vi "Lab Panel V4.83.vi"() -> ()   [LabVIEW 2013] (continued)
                            n2023 = local read "TDMS LAB02-2"() -> (w3251:refnum<k34>)
                            n2024 = Build Array(w3248) -> (w3243:dbl[])
                            n2025 = Build Array(w3246) -> (w3242:dbl[])
                            n2026 = Build Array(w3253) -> (w3241:dbl[])
                            n2027 = Build Array(w3254) -> (w3240:dbl[])
                            n2028 = Build Array(w3249) -> (w3245:dbl[])
                            n2029 = Build Array(w3247) -> (w3244:dbl[])
                            n2030 = Build Array(w3252) -> (w3239:dbl[])
                            n2031 = Build Array("AMPS ON", "AMPS OFF", "VOLTS", "PF", "TEMP Live", "TEMP Neut", "CYCLE") -> (w3222:string[])
                            n2032 = Bundle By Name("Y"=w3245, "t0"=w3238) -> (w3237:waveform(dbl))  [unwired: 1 in]
                            n2033 = Bundle By Name("Y"=w3244, "t0"=w3238) -> (w3236:waveform(dbl))  [unwired: 1 in]
                            n2034 = Bundle By Name("Y"=w3243, "t0"=w3238) -> (w3235:waveform(dbl))  [unwired: 1 in]
                            n2035 = Bundle By Name("Y"=w3242, "t0"=w3238) -> (w3234:waveform(dbl))  [unwired: 1 in]
                            n2036 = Bundle By Name("Y"=w3241, "t0"=w3238) -> (w3233:waveform(dbl))  [unwired: 1 in]
                            n2037 = Bundle By Name("Y"=w3240, "t0"=w3238) -> (w3232:waveform(dbl))  [unwired: 1 in]
                            n2038 = Bundle By Name("Y"=w3239, "t0"=w3238) -> (w3231:waveform(dbl))  [unwired: 1 in]
                            n2039 = Build Array(w3237, w3236, w3235, w3234, w3233, w3232, w3231) -> (w3230:waveform(dbl)[])
                            n2040 = TDMS Write(0:w3251, 5:"TEST VALUES", 7:w3222, 9:w3230) -> (4:w3221:refnum<k34>, 6:w3220:string, 15:w3219:errorcluster)  [unwired: 2 in, 1 out]
                            n2041 = TDMS Write(0:w3221, 5:w3220, 7:"TIME", 9:w3217, 11:w3219) -> (15:w3216:errorcluster)  [unwired: 1 in, 3 out]
                            n2042 = local write "data file error"(w3216) -> ()
                          }
                        }
                      }
                    }
                  }
                }
              }
              frame #4 {
                n2043 = case shown="True" w3255 {
                  tunnel: w3259 -> [_ w3264]
                  tunnel: w3258 -> [_ w3263]
                  tunnel: w3257 -> [_ w3261]
                  tunnel: w3256 -> [_ w3260]
                  frame False {
                  }
                  frame True {
                    n2044 = local read "DISP LAB03-1"() -> (w3265:T4)
                    n2045 = local read "SIG LAB03-1"() -> (w3266:T2)
                    n2046 = local read "ON L03-1"() -> (w3262:cluster{"amps":dbl, "volts":dbl, "pf":dbl})
                    n2047 = Unbundle(w3266) -> ("AMPS"=w3272:dbl, "VOLTS"=w3270:dbl, "PF"=w3269:dbl, "Tmp Live"=w3268:dbl, "Tmp Neut"=w3271:dbl)
                    n2048 = Unbundle(w3265) -> ("CYCLE"=w3267:dbl)  [unwired: 2 out]
                    n2049 = stacked-sequence {
                      tunnel: w3272 -> [w3276 w3295]
                      tunnel: w3271 -> [_ w3294]
                      tunnel: w3270 -> [w3275 w3293]
                      tunnel: w3269 -> [w3274 w3292]
                      tunnel: w3268 -> [_ w3291]
                      tunnel: w3267 -> [_ w3290]
                      tunnel: w3264 -> [_ w3289]
                      tunnel: w3263 -> [w3277 _]
                      tunnel: w3262 -> [w3273 w3287]
                      tunnel: w3261 -> [_ w3288]
                      tunnel: w3260 -> [_ w3283]
                      frame #0 {
                        n2050 = case shown="True" w3277 {
                          tunnel: w3276 -> [_ w3282]
                          tunnel: w3275 -> [_ w3281]
                          tunnel: w3274 -> [_ w3280]
                          tunnel: w3273 -> [_ w3278]
                          frame False {
                          }
                          frame True {
                            n2051 = Bundle(cluster=w3278, "amps"=w3282, "volts"=w3281, "pf"=w3280) -> (w3279:cluster{"amps":dbl, "volts":dbl, "pf":dbl})
                            n2052 = local write "ON L03-1"(w3279) -> ()
                          }
                        }
                      }
                      frame #1 {
                        n2053 = Unbundle(w3287) -> ("amps"=w3286:dbl, "volts"=w3285:dbl, "pf"=w3284:dbl)
                        n2054 = case shown="True" w3288 {
                          tunnel: w3295 -> [_ w3327]
                          tunnel: w3294 -> [_ w3334]
                          tunnel: w3293 -> [_ _]
                          tunnel: w3292 -> [_ _]
                          tunnel: w3291 -> [_ w3333]
                          tunnel: w3290 -> [_ w3332]
                          tunnel: w3289 -> [_ w3297]
                          tunnel: w3286 -> [_ w3329]
                          tunnel: w3285 -> [_ w3328]
                          tunnel: w3284 -> [_ w3326]
                          tunnel: w3283 -> [_ w3318]
                          frame False {
                          }
                          frame True {
                            n2055 = local read "TDMS LAB03-1"() -> (w3331:refnum<k34>)
                            n2056 = Build Array(w3328) -> (w3323:dbl[])
                            n2057 = Build Array(w3326) -> (w3322:dbl[])
                            n2058 = Build Array(w3333) -> (w3321:dbl[])
                            n2059 = Build Array(w3334) -> (w3320:dbl[])
                            n2060 = Build Array(w3329) -> (w3325:dbl[])
                            n2061 = Build Array(w3327) -> (w3324:dbl[])
                            n2062 = Build Array(w3332) -> (w3319:dbl[])
                            n2063 = Build Array("AMPS ON", "AMPS OFF", "VOLTS", "PF", "TEMP Live", "TEMP Neut", "CYCLE") -> (w3302:string[])
                            n2064 = Bundle By Name("Y"=w3325, "t0"=w3318) -> (w3317:waveform(dbl))  [unwired: 1 in]
                            n2065 = Bundle By Name("Y"=w3324, "t0"=w3318) -> (w3316:waveform(dbl))  [unwired: 1 in]
                            n2066 = Bundle By Name("Y"=w3323, "t0"=w3318) -> (w3315:waveform(dbl))  [unwired: 1 in]
                            n2067 = Bundle By Name("Y"=w3322, "t0"=w3318) -> (w3314:waveform(dbl))  [unwired: 1 in]
                            n2068 = Bundle By Name("Y"=w3321, "t0"=w3318) -> (w3313:waveform(dbl))  [unwired: 1 in]
                            n2069 = Bundle By Name("Y"=w3320, "t0"=w3318) -> (w3312:waveform(dbl))  [unwired: 1 in]
                            n2070 = Bundle By Name("Y"=w3319, "t0"=w3318) -> (w3311:waveform(dbl))  [unwired: 1 in]
                            n2071 = Build Array(w3317, w3316, w3315, w3314, w3313, w3312, w3311) -> (w3310:waveform(dbl)[])
                            n2072 = TDMS Write(0:w3331, 5:"TEST VALUES", 7:w3302, 9:w3310) -> (4:w3301:refnum<k34>, 6:w3300:string, 15:w3299:errorcluster)  [unwired: 2 in, 1 out]
                            n2073 = TDMS Write(0:w3301, 5:w3300, 7:"TIME", 9:w3297, 11:w3299) -> (15:w3296:errorcluster)  [unwired: 1 in, 3 out]
                            n2074 = local write "data file error"(w3296) -> ()
                          }
                        }
                      }
                    }
                  }
                }
              }
              frame #5 {
                n2075 = case shown="True" w3335 {
                  tunnel: w3339 -> [_ w3344]
                  tunnel: w3338 -> [_ w3343]
                  tunnel: w3337 -> [_ w3341]
                  tunnel: w3336 -> [_ w3340]
                  frame False {
                  }
                  frame True {
                    n2076 = local read "DISP LAB03-2"() -> (w3345:T4)
                    n2077 = local read "SIG LAB03-2"() -> (w3346:T2)
                    n2078 = local read "ON L03-2"() -> (w3342:cluster{"amps":dbl, "volts":dbl, "pf":dbl})
                    n2079 = Unbundle(w3346) -> ("AMPS"=w3352:dbl, "VOLTS"=w3350:dbl, "PF"=w3349:dbl, "Tmp Live"=w3348:dbl, "Tmp Neut"=w3351:dbl)
                    n2080 = Unbundle(w3345) -> ("CYCLE"=w3347:dbl)  [unwired: 2 out]
                    n2081 = stacked-sequence {
                      tunnel: w3352 -> [w3356 w3375]
                      tunnel: w3351 -> [_ w3374]
                      tunnel: w3350 -> [w3355 w3373]
                      tunnel: w3349 -> [w3354 w3372]
                      tunnel: w3348 -> [_ w3371]
                      tunnel: w3347 -> [_ w3370]
                      tunnel: w3344 -> [_ w3369]
                      tunnel: w3343 -> [w3357 _]
                      tunnel: w3342 -> [w3353 w3367]
                      tunnel: w3341 -> [_ w3368]
                      tunnel: w3340 -> [_ w3363]
                      frame #0 {
                        n2082 = case shown="True" w3357 {
                          tunnel: w3356 -> [_ w3362]
                          tunnel: w3355 -> [_ w3361]
                          tunnel: w3354 -> [_ w3360]
                          tunnel: w3353 -> [_ w3358]
                          frame False {
                          }
                          frame True {
                            n2083 = Bundle(cluster=w3358, "amps"=w3362, "volts"=w3361, "pf"=w3360) -> (w3359:cluster{"amps":dbl, "volts":dbl, "pf":dbl})
                            n2084 = local write "ON L03-2"(w3359) -> ()
                          }
                        }
                      }
                      frame #1 {
                        n2085 = Unbundle(w3367) -> ("amps"=w3366:dbl, "volts"=w3365:dbl, "pf"=w3364:dbl)
                        n2086 = case shown="True" w3368 {
                          tunnel: w3375 -> [_ w3407]
                          tunnel: w3374 -> [_ w3414]
                          tunnel: w3373 -> [_ _]
                          tunnel: w3372 -> [_ _]
                          tunnel: w3371 -> [_ w3413]
                          tunnel: w3370 -> [_ w3412]
                          tunnel: w3369 -> [_ w3377]
                          tunnel: w3366 -> [_ w3409]
                          tunnel: w3365 -> [_ w3408]
                          tunnel: w3364 -> [_ w3406]
                          tunnel: w3363 -> [_ w3398]
                          frame False {
                          }
                          frame True {
                            n2087 = local read "TDMS LAB03-2"() -> (w3411:refnum<k34>)
                            n2088 = Build Array(w3408) -> (w3403:dbl[])
                            n2089 = Build Array(w3406) -> (w3402:dbl[])
                            n2090 = Build Array(w3413) -> (w3401:dbl[])
                            n2091 = Build Array(w3414) -> (w3400:dbl[])
                            n2092 = Build Array(w3409) -> (w3405:dbl[])
                            n2093 = Build Array(w3407) -> (w3404:dbl[])
                            n2094 = Build Array(w3412) -> (w3399:dbl[])
                            n2095 = Build Array("AMPS ON", "AMPS OFF", "VOLTS", "PF", "TEMP Live", "TEMP Neut", "CYCLE") -> (w3382:string[])
                            n2096 = Bundle By Name("Y"=w3405, "t0"=w3398) -> (w3397:waveform(dbl))  [unwired: 1 in]
                            n2097 = Bundle By Name("Y"=w3404, "t0"=w3398) -> (w3396:waveform(dbl))  [unwired: 1 in]
                            n2098 = Bundle By Name("Y"=w3403, "t0"=w3398) -> (w3395:waveform(dbl))  [unwired: 1 in]
                            n2099 = Bundle By Name("Y"=w3402, "t0"=w3398) -> (w3394:waveform(dbl))  [unwired: 1 in]
                            n2100 = Bundle By Name("Y"=w3401, "t0"=w3398) -> (w3393:waveform(dbl))  [unwired: 1 in]
                            n2101 = Bundle By Name("Y"=w3400, "t0"=w3398) -> (w3392:waveform(dbl))  [unwired: 1 in]
                            n2102 = Bundle By Name("Y"=w3399, "t0"=w3398) -> (w3391:waveform(dbl))  [unwired: 1 in]
                            n2103 = Build Array(w3397, w3396, w3395, w3394, w3393, w3392, w3391) -> (w3390:waveform(dbl)[])
                            n2104 = TDMS Write(0:w3411, 5:"TEST VALUES", 7:w3382, 9:w3390) -> (4:w3381:refnum<k34>, 6:w3380:string, 15:w3379:errorcluster)  [unwired: 2 in, 1 out]
                            n2105 = TDMS Write(0:w3381, 5:w3380, 7:"TIME", 9:w3377, 11:w3379) -> (15:w3376:errorcluster)  [unwired: 1 in, 3 out]
                            n2106 = local write "data file error"(w3376) -> ()
                          }
                        }
                      }
                    }
                  }
                }
              }
              frame #6 {
                n2107 = case shown="True" w3415 {
                  tunnel: w3419 -> [_ w3424]
                  tunnel: w3418 -> [_ w3423]
                  tunnel: w3417 -> [_ w3421]
                  tunnel: w3416 -> [_ w3420]
                  frame False {
                  }
                  frame True {
                    n2108 = local read "DISP LAB04-1"() -> (w3425:T4)
                    n2109 = local read "SIG LAB04-1"() -> (w3426:T2)
                    n2110 = local read "ON L04-1"() -> (w3422:cluster{"amps":dbl, "volts":dbl, "pf":dbl})
                    n2111 = Unbundle(w3426) -> ("AMPS"=w3432:dbl, "VOLTS"=w3430:dbl, "PF"=w3429:dbl, "Tmp Live"=w3428:dbl, "Tmp Neut"=w3431:dbl)
                    n2112 = Unbundle(w3425) -> ("CYCLE"=w3427:dbl)  [unwired: 2 out]
                    n2113 = stacked-sequence {
                      tunnel: w3432 -> [w3436 w3455]
                      tunnel: w3431 -> [_ w3454]
                      tunnel: w3430 -> [w3435 w3453]
                      tunnel: w3429 -> [w3434 w3452]
                      tunnel: w3428 -> [_ w3451]
                      tunnel: w3427 -> [_ w3450]
                      tunnel: w3424 -> [_ w3449]
                      tunnel: w3423 -> [w3437 _]
                      tunnel: w3422 -> [w3433 w3447]
                      tunnel: w3421 -> [_ w3448]
                      tunnel: w3420 -> [_ w3443]
                      frame #0 {
                        n2114 = case shown="True" w3437 {
                          tunnel: w3436 -> [_ w3442]
                          tunnel: w3435 -> [_ w3441]
                          tunnel: w3434 -> [_ w3440]
                          tunnel: w3433 -> [_ w3438]
                          frame False {
                          }
                          frame True {
                            n2115 = Bundle(cluster=w3438, "amps"=w3442, "volts"=w3441, "pf"=w3440) -> (w3439:cluster{"amps":dbl, "volts":dbl, "pf":dbl})
                            n2116 = local write "ON L04-1"(w3439) -> ()
                          }
                        }
                      }
                      frame #1 {
                        n2117 = Unbundle(w3447) -> ("amps"=w3446:dbl, "volts"=w3445:dbl, "pf"=w3444:dbl)
                        n2118 = case shown="True" w3448 {
                          tunnel: w3455 -> [_ w3487]
                          tunnel: w3454 -> [_ w3494]
                          tunnel: w3453 -> [_ _]
                          tunnel: w3452 -> [_ _]
                          tunnel: w3451 -> [_ w3493]
                          tunnel: w3450 -> [_ w3492]
                          tunnel: w3449 -> [_ w3457]
                          tunnel: w3446 -> [_ w3489]
                          tunnel: w3445 -> [_ w3488]
                          tunnel: w3444 -> [_ w3486]
                          tunnel: w3443 -> [_ w3478]
                          frame False {
                          }
                          frame True {
                            n2119 = local read "TDMS LAB04-1"() -> (w3491:refnum<k34>)
                            n2120 = Build Array(w3488) -> (w3483:dbl[])
                            n2121 = Build Array(w3486) -> (w3482:dbl[])
                            n2122 = Build Array(w3493) -> (w3481:dbl[])
                            n2123 = Build Array(w3494) -> (w3480:dbl[])
                            n2124 = Build Array(w3489) -> (w3485:dbl[])
                            n2125 = Build Array(w3487) -> (w3484:dbl[])
                            n2126 = Build Array(w3492) -> (w3479:dbl[])
                            n2127 = Build Array("AMPS ON", "AMPS OFF", "VOLTS", "PF", "TEMP Live", "TEMP Neut", "CYCLE") -> (w3462:string[])
                            n2128 = Bundle By Name("Y"=w3485, "t0"=w3478) -> (w3477:waveform(dbl))  [unwired: 1 in]
                            n2129 = Bundle By Name("Y"=w3484, "t0"=w3478) -> (w3476:waveform(dbl))  [unwired: 1 in]
                            n2130 = Bundle By Name("Y"=w3483, "t0"=w3478) -> (w3475:waveform(dbl))  [unwired: 1 in]
                            n2131 = Bundle By Name("Y"=w3482, "t0"=w3478) -> (w3474:waveform(dbl))  [unwired: 1 in]
                            n2132 = Bundle By Name("Y"=w3481, "t0"=w3478) -> (w3473:waveform(dbl))  [unwired: 1 in]
                            n2133 = Bundle By Name("Y"=w3480, "t0"=w3478) -> (w3472:waveform(dbl))  [unwired: 1 in]
                            n2134 = Bundle By Name("Y"=w3479, "t0"=w3478) -> (w3471:waveform(dbl))  [unwired: 1 in]
                            n2135 = Build Array(w3477, w3476, w3475, w3474, w3473, w3472, w3471) -> (w3470:waveform(dbl)[])
                            n2136 = TDMS Write(0:w3491, 5:"TEST VALUES", 7:w3462, 9:w3470) -> (4:w3461:refnum<k34>, 6:w3460:string, 15:w3459:errorcluster)  [unwired: 2 in, 1 out]
                            n2137 = TDMS Write(0:w3461, 5:w3460, 7:"TIME", 9:w3457, 11:w3459) -> (15:w3456:errorcluster)  [unwired: 1 in, 3 out]
                            n2138 = local write "data file error"(w3456) -> ()
                          }
                        }
                      }
                    }
                  }
                }
              }
              frame #7 {
                n2139 = case shown="True" w3495 {
                  tunnel: w3499 -> [_ w3504]
                  tunnel: w3498 -> [_ w3503]
                  tunnel: w3497 -> [_ w3501]
                  tunnel: w3496 -> [_ w3500]
                  frame False {
                  }
                  frame True {
                    n2140 = local read "DISP LAB04-2"() -> (w3505:T4)
                    n2141 = local read "SIG LAB04-2"() -> (w3506:T2)
                    n2142 = local read "ON L04-2"() -> (w3502:cluster{"amps":dbl, "volts":dbl, "pf":dbl})
                    n2143 = Unbundle(w3506) -> ("AMPS"=w3512:dbl, "VOLTS"=w3510:dbl, "PF"=w3509:dbl, "Tmp Live"=w3508:dbl, "Tmp Neut"=w3511:dbl)
                    n2144 = Unbundle(w3505) -> ("CYCLE"=w3507:dbl)  [unwired: 2 out]
                    n2145 = stacked-sequence {
                      tunnel: w3512 -> [w3516 w3535]
                      tunnel: w3511 -> [_ w3534]
                      tunnel: w3510 -> [w3515 w3533]
                      tunnel: w3509 -> [w3514 w3532]
                      tunnel: w3508 -> [_ w3531]
                      tunnel: w3507 -> [_ w3530]
                      tunnel: w3504 -> [_ w3529]
                      tunnel: w3503 -> [w3517 _]
                      tunnel: w3502 -> [w3513 w3527]
                      tunnel: w3501 -> [_ w3528]
                      tunnel: w3500 -> [_ w3523]
                      frame #0 {
                        n2146 = case shown="True" w3517 {
                          tunnel: w3516 -> [_ w3522]
                          tunnel: w3515 -> [_ w3521]
                          tunnel: w3514 -> [_ w3520]
                          tunnel: w3513 -> [_ w3518]
                          frame False {
                          }
                          frame True {
                            n2147 = Bundle(cluster=w3518, "amps"=w3522, "volts"=w3521, "pf"=w3520) -> (w3519:cluster{"amps":dbl, "volts":dbl, "pf":dbl})
                            n2148 = local write "ON L04-2"(w3519) -> ()
                          }
                        }
                      }
                      frame #1 {
                        n2149 = Unbundle(w3527) -> ("amps"=w3526:dbl, "volts"=w3525:dbl, "pf"=w3524:dbl)
                        n2150 = case shown="True" w3528 {
                          tunnel: w3535 -> [_ w3567]
                          tunnel: w3534 -> [_ w3574]
                          tunnel: w3533 -> [_ _]
                          tunnel: w3532 -> [_ _]
                          tunnel: w3531 -> [_ w3573]
                          tunnel: w3530 -> [_ w3572]
                          tunnel: w3529 -> [_ w3537]
                          tunnel: w3526 -> [_ w3569]
                          tunnel: w3525 -> [_ w3568]
                          tunnel: w3524 -> [_ w3566]
                          tunnel: w3523 -> [_ w3558]
                          frame False {
                          }
                          frame True {
                            n2151 = local read "TDMS LAB04-2"() -> (w3571:refnum<k34>)
                            n2152 = Build Array(w3568) -> (w3563:dbl[])
                            n2153 = Build Array(w3566) -> (w3562:dbl[])
                            n2154 = Build Array(w3573) -> (w3561:dbl[])
                            n2155 = Build Array(w3574) -> (w3560:dbl[])
                            n2156 = Build Array(w3569) -> (w3565:dbl[])
                            n2157 = Build Array(w3567) -> (w3564:dbl[])
                            n2158 = Build Array(w3572) -> (w3559:dbl[])
                            n2159 = Build Array("AMPS ON", "AMPS OFF", "VOLTS", "PF", "TEMP Live", "TEMP Neut", "CYCLE") -> (w3542:string[])
                            n2160 = Bundle By Name("Y"=w3565, "t0"=w3558) -> (w3557:waveform(dbl))  [unwired: 1 in]
                            n2161 = Bundle By Name("Y"=w3564, "t0"=w3558) -> (w3556:waveform(dbl))  [unwired: 1 in]
                            n2162 = Bundle By Name("Y"=w3563, "t0"=w3558) -> (w3555:waveform(dbl))  [unwired: 1 in]
                            n2163 = Bundle By Name("Y"=w3562, "t0"=w3558) -> (w3554:waveform(dbl))  [unwired: 1 in]
                            n2164 = Bundle By Name("Y"=w3561, "t0"=w3558) -> (w3553:waveform(dbl))  [unwired: 1 in]
                            n2165 = Bundle By Name("Y"=w3560, "t0"=w3558) -> (w3552:waveform(dbl))  [unwired: 1 in]
                            n2166 = Bundle By Name("Y"=w3559, "t0"=w3558) -> (w3551:waveform(dbl))  [unwired: 1 in]
                            n2167 = Build Array(w3557, w3556, w3555, w3554, w3553, w3552, w3551) -> (w3550:waveform(dbl)[])
                            n2168 = TDMS Write(0:w3571, 5:"TEST VALUES", 7:w3542, 9:w3550) -> (4:w3541:refnum<k34>, 6:w3540:string, 15:w3539:errorcluster)  [unwired: 2 in, 1 out]
                            n2169 = TDMS Write(0:w3541, 5:w3540, 7:"TIME", 9:w3537, 11:w3539) -> (15:w3536:errorcluster)  [unwired: 1 in, 3 out]
                            n2170 = local write "data file error"(w3536) -> ()
                          }
                        }
                      }
                    }
                  }
                }
              }
              frame #8 {
                n2171 = case shown="True" w3575 {
                  tunnel: w3579 -> [_ w3584]
                  tunnel: w3578 -> [_ w3583]
                  tunnel: w3577 -> [_ w3581]
                  tunnel: w3576 -> [_ w3580]
                  frame False {
                  }
                  frame True {
                    n2172 = local read "DISP LAB05-1"() -> (w3585:T4)
                    n2173 = local read "SIG LAB05-1"() -> (w3586:T2)
                    n2174 = local read "ON L05-1"() -> (w3582:cluster{"amps":dbl, "volts":dbl, "pf":dbl})
                    n2175 = Unbundle(w3586) -> ("AMPS"=w3592:dbl, "VOLTS"=w3590:dbl, "PF"=w3589:dbl, "Tmp Live"=w3588:dbl, "Tmp Neut"=w3591:dbl)
                    n2176 = Unbundle(w3585) -> ("CYCLE"=w3587:dbl)  [unwired: 2 out]
                    n2177 = stacked-sequence {
                      tunnel: w3592 -> [w3596 w3615]
                      tunnel: w3591 -> [_ w3614]
                      tunnel: w3590 -> [w3595 w3613]
                      tunnel: w3589 -> [w3594 w3612]
                      tunnel: w3588 -> [_ w3611]
                      tunnel: w3587 -> [_ w3610]
                      tunnel: w3584 -> [_ w3609]
                      tunnel: w3583 -> [w3597 _]
                      tunnel: w3582 -> [w3593 w3607]
                      tunnel: w3581 -> [_ w3608]
                      tunnel: w3580 -> [_ w3603]
                      frame #0 {
                        n2178 = case shown="True" w3597 {
                          tunnel: w3596 -> [_ w3602]
                          tunnel: w3595 -> [_ w3601]
                          tunnel: w3594 -> [_ w3600]
                          tunnel: w3593 -> [_ w3598]
                          frame False {
                          }
                          frame True {
                            n2179 = Bundle(cluster=w3598, "amps"=w3602, "volts"=w3601, "pf"=w3600) -> (w3599:cluster{"amps":dbl, "volts":dbl, "pf":dbl})
                            n2180 = local write "ON L05-1"(w3599) -> ()
                          }
                        }
                      }
                      frame #1 {
                        n2181 = Unbundle(w3607) -> ("amps"=w3606:dbl, "volts"=w3605:dbl, "pf"=w3604:dbl)
                        n2182 = case shown="True" w3608 {
                          tunnel: w3615 -> [_ w3647]
                          tunnel: w3614 -> [_ w3654]
                          tunnel: w3613 -> [_ _]
                          tunnel: w3612 -> [_ _]
                          tunnel: w3611 -> [_ w3653]
                          tunnel: w3610 -> [_ w3652]
                          tunnel: w3609 -> [_ w3617]
                          tunnel: w3606 -> [_ w3649]
                          tunnel: w3605 -> [_ w3648]
                          tunnel: w3604 -> [_ w3646]
                          tunnel: w3603 -> [_ w3638]
                          frame False {
                          }
                          frame True {
                            n2183 = local read "TDMS LAB05-1"() -> (w3651:refnum<k34>)
                            n2184 = Build Array(w3648) -> (w3643:dbl[])
                            n2185 = Build Array(w3646) -> (w3642:dbl[])
                            n2186 = Build Array(w3653) -> (w3641:dbl[])
                            n2187 = Build Array(w3654) -> (w3640:dbl[])
                            n2188 = Build Array(w3649) -> (w3645:dbl[])
                            n2189 = Build Array(w3647) -> (w3644:dbl[])
                            n2190 = Build Array(w3652) -> (w3639:dbl[])
                            n2191 = Build Array("AMPS ON", "AMPS OFF", "VOLTS", "PF", "TEMP Live", "TEMP Neut", "CYCLE") -> (w3622:string[])
                            n2192 = Bundle By Name("Y"=w3645, "t0"=w3638) -> (w3637:waveform(dbl))  [unwired: 1 in]
                            n2193 = Bundle By Name("Y"=w3644, "t0"=w3638) -> (w3636:waveform(dbl))  [unwired: 1 in]
                            n2194 = Bundle By Name("Y"=w3643, "t0"=w3638) -> (w3635:waveform(dbl))  [unwired: 1 in]
                            n2195 = Bundle By Name("Y"=w3642, "t0"=w3638) -> (w3634:waveform(dbl))  [unwired: 1 in]
                            n2196 = Bundle By Name("Y"=w3641, "t0"=w3638) -> (w3633:waveform(dbl))  [unwired: 1 in]
                            n2197 = Bundle By Name("Y"=w3640, "t0"=w3638) -> (w3632:waveform(dbl))  [unwired: 1 in]
                            n2198 = Bundle By Name("Y"=w3639, "t0"=w3638) -> (w3631:waveform(dbl))  [unwired: 1 in]
                            n2199 = Build Array(w3637, w3636, w3635, w3634, w3633, w3632, w3631) -> (w3630:waveform(dbl)[])
                            n2200 = TDMS Write(0:w3651, 5:"TEST VALUES", 7:w3622, 9:w3630) -> (4:w3621:refnum<k34>, 6:w3620:string, 15:w3619:errorcluster)  [unwired: 2 in, 1 out]
                            n2201 = TDMS Write(0:w3621, 5:w3620, 7:"TIME", 9:w3617, 11:w3619) -> (15:w3616:errorcluster)  [unwired: 1 in, 3 out]
                            n2202 = local write "data file error"(w3616) -> ()
                          }
                        }
                      }
                    }
                  }
                }
              }
              frame #9 {
                n2203 = case shown="True" w3655 {
                  tunnel: w3659 -> [_ w3664]
                  tunnel: w3658 -> [_ w3663]
                  tunnel: w3657 -> [_ w3661]
                  tunnel: w3656 -> [_ w3660]
                  frame False {
                  }
                  frame True {
                    n2204 = local read "DISP LAB05-2"() -> (w3665:T4)
                    n2205 = local read "SIG LAB05-2"() -> (w3666:T2)
                    n2206 = local read "ON L05-2"() -> (w3662:cluster{"amps":dbl, "volts":dbl, "pf":dbl})
                    n2207 = Unbundle(w3666) -> ("AMPS"=w3672:dbl, "VOLTS"=w3670:dbl, "PF"=w3669:dbl, "Tmp Live"=w3668:dbl, "Tmp Neut"=w3671:dbl)
                    n2208 = Unbundle(w3665) -> ("CYCLE"=w3667:dbl)  [unwired: 2 out]
                    n2209 = stacked-sequence {
                      tunnel: w3672 -> [w3676 w3695]
                      tunnel: w3671 -> [_ w3694]
                      tunnel: w3670 -> [w3675 w3693]
                      tunnel: w3669 -> [w3674 w3692]
                      tunnel: w3668 -> [_ w3691]
                      tunnel: w3667 -> [_ w3690]
                      tunnel: w3664 -> [_ w3689]
                      tunnel: w3663 -> [w3677 _]
                      tunnel: w3662 -> [w3673 w3687]
                      tunnel: w3661 -> [_ w3688]
                      tunnel: w3660 -> [_ w3683]
                      frame #0 {
                        n2210 = case shown="True" w3677 {
                          tunnel: w3676 -> [_ w3682]
                          tunnel: w3675 -> [_ w3681]
                          tunnel: w3674 -> [_ w3680]
                          tunnel: w3673 -> [_ w3678]
                          frame False {
                          }
                          frame True {
                            n2211 = Bundle(cluster=w3678, "amps"=w3682, "volts"=w3681, "pf"=w3680) -> (w3679:cluster{"amps":dbl, "volts":dbl, "pf":dbl})
                            n2212 = local write "ON L05-2"(w3679) -> ()
                          }
                        }
                      }
                      frame #1 {
                        n2213 = Unbundle(w3687) -> ("amps"=w3686:dbl, "volts"=w3685:dbl, "pf"=w3684:dbl)
                        n2214 = case shown="True" w3688 {
                          tunnel: w3695 -> [_ w3727]
                          tunnel: w3694 -> [_ w3734]
                          tunnel: w3693 -> [_ _]
                          tunnel: w3692 -> [_ _]
                          tunnel: w3691 -> [_ w3733]
                          tunnel: w3690 -> [_ w3732]
                          tunnel: w3689 -> [_ w3697]
                          tunnel: w3686 -> [_ w3729]
                          tunnel: w3685 -> [_ w3728]
                          tunnel: w3684 -> [_ w3726]
                          tunnel: w3683 -> [_ w3718]
                          frame False {
                          }
                          frame True {
                            n2215 = local read "TDMS LAB05-2"() -> (w3731:refnum<k34>)
                            n2216 = Build Array(w3728) -> (w3723:dbl[])
                            n2217 = Build Array(w3726) -> (w3722:dbl[])
                            n2218 = Build Array(w3733) -> (w3721:dbl[])
                            n2219 = Build Array(w3734) -> (w3720:dbl[])
                            n2220 = Build Array(w3729) -> (w3725:dbl[])
                            n2221 = Build Array(w3727) -> (w3724:dbl[])
                            n2222 = Build Array(w3732) -> (w3719:dbl[])
                            n2223 = Build Array("AMPS ON", "AMPS OFF", "VOLTS", "PF", "TEMP Live", "TEMP Neut", "CYCLE") -> (w3702:string[])
                            n2224 = Bundle By Name("Y"=w3725, "t0"=w3718) -> (w3717:waveform(dbl))  [unwired: 1 in]
                            n2225 = Bundle By Name("Y"=w3724, "t0"=w3718) -> (w3716:waveform(dbl))  [unwired: 1 in]
                            n2226 = Bundle By Name("Y"=w3723, "t0"=w3718) -> (w3715:waveform(dbl))  [unwired: 1 in]
                            n2227 = Bundle By Name("Y"=w3722, "t0"=w3718) -> (w3714:waveform(dbl))  [unwired: 1 in]
                            n2228 = Bundle By Name("Y"=w3721, "t0"=w3718) -> (w3713:waveform(dbl))  [unwired: 1 in]
                            n2229 = Bundle By Name("Y"=w3720, "t0"=w3718) -> (w3712:waveform(dbl))  [unwired: 1 in]
                            n2230 = Bundle By Name("Y"=w3719, "t0"=w3718) -> (w3711:waveform(dbl))  [unwired: 1 in]
                            n2231 = Build Array(w3717, w3716, w3715, w3714, w3713, w3712, w3711) -> (w3710:waveform(dbl)[])
                            n2232 = TDMS Write(0:w3731, 5:"TEST VALUES", 7:w3702, 9:w3710) -> (4:w3701:refnum<k34>, 6:w3700:string, 15:w3699:errorcluster)  [unwired: 2 in, 1 out]
                            n2233 = TDMS Write(0:w3701, 5:w3700, 7:"TIME", 9:w3697, 11:w3699) -> (15:w3696:errorcluster)  [unwired: 1 in, 3 out]
                            n2234 = local write "data file error"(w3696) -> ()
                          }
                        }
                      }
                    }
                  }
                }
              }
            }
          }
          frame #13 {
            # "display test values on chart"
            n2235 = case shown="\"OFF CYCLE\"" "Select  Cycle" {
              tunnel: [1 w3740] -> w3736
              frame "ON CYCLE", Default {
              }
              frame "OFF CYCLE" {
                n2236 = local read "on loops"() -> (w3742:dbl)
                n2237 = Add(x=w3742, y=2) -> (x+y=w3740:dbl)
              }
            }
            n2238 = local read "jig cycle"() -> (w3738:dbl)
            n2239 = Equal?(x=w3738, y=w3736) -> (x = y?=w3735:bool)
            "graph flag" <- w3735
            n2240 = global write "Global display 3.vi" "graph flag"(w3735) -> ()
            n2241 = case shown="True" w3735 {
              frame False {
              }
              frame True {
                n2242 = local read "SIG LAB05-1"() -> (w3784:T2)
                n2243 = local read "SIG LAB04-2"() -> (w3785:T2)
                n2244 = local read "SIG LAB05-2"() -> (w3783:T2)
                n2245 = local read "SIG LAB04-1"() -> (w3786:T2)
                n2246 = local read "SIG LAB03-1"() -> (w3788:T2)
                n2247 = local read "SIG LAB03-2"() -> (w3787:T2)
                n2248 = local read "SIG LAB01-1"() -> (w3792:T2)
                n2249 = local read "SIG LAB02-2"() -> (w3789:T2)
                n2250 = local read "SIG LAB02-1"() -> (w3790:T2)
                n2251 = local read "SIG LAB01-2"() -> (w3791:T2)
                n2252 = Unbundle(w3785) -> ("AMPS"=w3775:dbl, "VOLTS"=w3765:dbl, "Tmp Live"=w3755:dbl, "Tmp Neut"=w3745:dbl)  [unwired: 1 out]
                n2253 = Unbundle(w3784) -> ("AMPS"=w3774:dbl, "VOLTS"=w3764:dbl, "Tmp Live"=w3754:dbl, "Tmp Neut"=w3744:dbl)  [unwired: 1 out]
                n2254 = Unbundle(w3783) -> ("AMPS"=w3773:dbl, "VOLTS"=w3763:dbl, "Tmp Live"=w3753:dbl, "Tmp Neut"=w3743:dbl)  [unwired: 1 out]
                n2255 = Unbundle(w3786) -> ("AMPS"=w3776:dbl, "VOLTS"=w3766:dbl, "Tmp Live"=w3756:dbl, "Tmp Neut"=w3746:dbl)  [unwired: 1 out]
                n2256 = Unbundle(w3787) -> ("AMPS"=w3777:dbl, "VOLTS"=w3767:dbl, "Tmp Live"=w3757:dbl, "Tmp Neut"=w3747:dbl)  [unwired: 1 out]
                n2257 = Unbundle(w3788) -> ("AMPS"=w3778:dbl, "VOLTS"=w3768:dbl, "Tmp Live"=w3758:dbl, "Tmp Neut"=w3748:dbl)  [unwired: 1 out]
                n2258 = Unbundle(w3789) -> ("AMPS"=w3779:dbl, "VOLTS"=w3769:dbl, "Tmp Live"=w3759:dbl, "Tmp Neut"=w3749:dbl)  [unwired: 1 out]
                n2259 = Unbundle(w3790) -> ("AMPS"=w3780:dbl, "VOLTS"=w3770:dbl, "Tmp Live"=w3760:dbl, "Tmp Neut"=w3750:dbl)  [unwired: 1 out]
                n2260 = Unbundle(w3792) -> ("AMPS"=w3782:dbl, "VOLTS"=w3772:dbl, "Tmp Live"=w3762:dbl, "Tmp Neut"=w3752:dbl)  [unwired: 1 out]
                n2261 = Unbundle(w3791) -> ("AMPS"=w3781:dbl, "VOLTS"=w3771:dbl, "Tmp Live"=w3761:dbl, "Tmp Neut"=w3751:dbl)  [unwired: 1 out]
                n2262 = stacked-sequence {
                  tunnel: w3782 -> [w3803 _ _ _ _]
                  tunnel: w3781 -> [w3802 _ _ _ _]
                  tunnel: w3780 -> [w3801 _ _ _ _]
                  tunnel: w3779 -> [w3800 _ _ _ _]
                  tunnel: w3778 -> [w3799 _ _ _ _]
                  tunnel: w3777 -> [w3798 _ _ _ _]
                  tunnel: w3776 -> [w3797 _ _ _ _]
                  tunnel: w3775 -> [w3796 _ _ _ _]
                  tunnel: w3774 -> [w3795 _ _ _ _]
                  tunnel: w3773 -> [w3794 _ _ _ _]
                  tunnel: w3772 -> [_ w3814 _ _ _]
                  tunnel: w3771 -> [_ w3813 _ _ _]
                  tunnel: w3770 -> [_ w3812 _ _ _]
                  tunnel: w3769 -> [_ w3811 _ _ _]
                  tunnel: w3768 -> [_ w3810 _ _ _]
                  tunnel: w3767 -> [_ w3809 _ _ _]
                  tunnel: w3766 -> [_ w3808 _ _ _]
                  tunnel: w3765 -> [_ w3807 _ _ _]
                  tunnel: w3764 -> [_ w3806 _ _ _]
                  tunnel: w3763 -> [_ w3805 _ _ _]
                  tunnel: w3762 -> [_ _ w3825 _ _]
                  tunnel: w3761 -> [_ _ w3824 _ _]
                  tunnel: w3760 -> [_ _ w3823 _ _]
                  tunnel: w3759 -> [_ _ w3822 _ _]
                  tunnel: w3758 -> [_ _ w3821 _ _]
                  tunnel: w3757 -> [_ _ w3820 _ _]
                  tunnel: w3756 -> [_ _ w3819 _ _]
                  tunnel: w3755 -> [_ _ w3818 _ _]
                  tunnel: w3754 -> [_ _ w3817 _ _]
                  tunnel: w3753 -> [_ _ w3816 _ _]
                  tunnel: w3752 -> [_ _ _ w3836 _]
                  tunnel: w3751 -> [_ _ _ w3835 _]
                  tunnel: w3750 -> [_ _ _ w3834 _]
                  tunnel: w3749 -> [_ _ _ w3833 _]
                  tunnel: w3748 -> [_ _ _ w3832 _]
                  tunnel: w3747 -> [_ _ _ w3831 _]
                  tunnel: w3746 -> [_ _ _ w3830 _]
                  tunnel: w3745 -> [_ _ _ w3829 _]
                  tunnel: w3744 -> [_ _ _ w3828 _]
                  tunnel: w3743 -> [_ _ _ w3827 _]
                  frame #0 {
                    n2263 = Merge Signals(w3803, w3802, w3801, w3800, w3799, w3798, w3797, w3796, w3795, w3794) -> (→"TEST AMPS CHART":dynamicdata)
                  }
                  frame #1 {
                    n2264 = Merge Signals(w3814, w3813, w3812, w3811, w3810, w3809, w3808, w3807, w3806, w3805) -> (→"TEST VOLTS CHART":dynamicdata)
                  }
                  frame #2 {
                    n2265 = Merge Signals(w3825, w3824, w3823, w3822, w3821, w3820, w3819, w3818, w3817, w3816) -> (→"TEMPERATURE (L) CHART":dynamicdata)
                  }
                  frame #3 {
                    n2266 = Merge Signals(w3836, w3835, w3834, w3833, w3832, w3831, w3830, w3829, w3828, w3827) -> (→"TEMPERATURE (N) CHART":dynamicdata)
                  }
                  frame #4 {
                    n2267 = local read "TEMPERATURE (N) CHART"() -> (w3837:dynamicdata)
                    n2268 = local read "TEMPERATURE (L) CHART"() -> (w3838:dynamicdata)
                    n2269 = local read "TEST VOLTS CHART"() -> (w3839:dynamicdata)
                    n2270 = local read "TEST AMPS CHART"() -> (w3840:dynamicdata)
                    n2271 = global write "Global display 3.vi" "graph temp N"(w3837) -> ()
                    n2272 = global write "Global display 3.vi" "graph temp L"(w3838) -> ()
                    n2273 = global write "Global display 3.vi" "graph volts"(w3839) -> ()
                    n2274 = global write "Global display 3.vi" "graph amps"(w3840) -> ()
                  }
                }
              }
            }
          }
          frame #14 {
            # "check for amps fail"
            # "check for cycle test & temperature rise fail conditions"
            n2275 = local read "on loops"() -> (w3867:dbl)
            n2276 = local read "jig cycle"() -> (w3864:dbl)
            n2277 = local read "jig cycle"() -> (w3869:dbl)
            n2278 = Add(x=w3867, y=3.0) -> (x+y=w3865:dbl)
            n2279 = Equal?(x=w3864, y=w3865) -> (x = y?=w3860:bool)
            n2280 = local read "Fail Loops"() -> (w3841:dbl)
            n2281 = Equal?(x=w3869, y=1.0) -> (x = y?=w3862:bool)
            n2282 = global write "Global 1.vi" "fail count"(w3841) -> ()
            n2283 = stacked-sequence {
              tunnel: w3863 -> [w3872 _ _ _ _ _ _ _ _ _]
              tunnel: w3862 -> [w3873 w3893 w3913 w3933 w3953 w3973 w3993 w4013 w4033 w4053]
              tunnel: w3861 -> [w3870 _ _ _ _ _ _ _ _ _]
              tunnel: w3860 -> [w3871 w3892 w3912 w3932 w3952 w3972 w3992 w4012 w4032 w4052]
              tunnel: w3859 -> [_ w3891 _ _ _ _ _ _ _ _]
              tunnel: w3858 -> [_ w3890 _ _ _ _ _ _ _ _]
              tunnel: w3857 -> [_ _ w3911 _ _ _ _ _ _ _]
              tunnel: w3856 -> [_ _ w3910 _ _ _ _ _ _ _]
              tunnel: w3855 -> [_ _ _ w3931 _ _ _ _ _ _]
              tunnel: w3854 -> [_ _ _ w3930 _ _ _ _ _ _]
              tunnel: w3853 -> [_ _ _ _ w3951 _ _ _ _ _]
              tunnel: w3852 -> [_ _ _ _ w3950 _ _ _ _ _]
              tunnel: w3851 -> [_ _ _ _ _ w3971 _ _ _ _]
              tunnel: w3850 -> [_ _ _ _ _ w3970 _ _ _ _]
              tunnel: w3849 -> [_ _ _ _ _ _ w3991 _ _ _]
              tunnel: w3848 -> [_ _ _ _ _ _ w3990 _ _ _]
              tunnel: w3847 -> [_ _ _ _ _ _ _ w4011 _ _]
              tunnel: w3846 -> [_ _ _ _ _ _ _ w4010 _ _]
              tunnel: w3845 -> [_ _ _ _ _ _ _ _ w4031 _]
              tunnel: w3844 -> [_ _ _ _ _ _ _ _ w4030 _]
              tunnel: w3843 -> [_ _ _ _ _ _ _ _ _ w4051]
              tunnel: w3842 -> [_ _ _ _ _ _ _ _ _ w4050]
              frame #0 {
                # "LAB01-1"
                n2284 = case shown="True" w3870 {
                  tunnel: w3873 -> [_ w3886]
                  tunnel: w3872 -> [_ w3883]
                  tunnel: w3871 -> [_ w3882]
                  frame False {
                  }
                  frame True {
                    n2285 = local read "TEMP START LAB01-1"() -> (w3888:cluster{"TL":dbl, "TN":dbl})
                    n2286 = local read "RESULT LAB01-1"() -> (w3877:bool)
                    n2287 = local read "FAIL LAB01-1"() -> (w3880:cluster{"LO":dbl, "HI":dbl})
                    n2288 = local read "TDMS LAB01-1"() -> (w3887:refnum<k34>)
                    n2289 = local read "SET LAB01-1"() -> (w3884:T5)
                    n2290 = local read "DISP LAB01-1"() -> (w3885:T4)
                    n2291 = local read "SIG LAB01-1"() -> (w3889:T2)
                    n2292 = Bundle("FAIL LAB01-1"=w3880, "SIG LAB01-1"=w3889, "TEMP START LAB01-1"=w3888, "DISP LAB01-1"=w3885, "SET LAB01-1"=w3884, "TDMS LAB01-1"=w3887) -> (w3874:T28)  [unwired: 1 in]
                    n2293 = call "sub vi - cycle&temp fail v6.vi"("Amps Lo?"=w3886, "Input Cluster"=w3874, "SELECT"=w3883, "Amps Hi?"=w3882, "Result In"=w3877) -> ("(FAIL) out"=w3879:cluster{"FAIL LO":dbl, "FAIL HI":dbl}, "(DISP) out"=w3875:T4, "T-RISE"=w3876:cluster{"T-RISE (L)":dbl, "T-RISE (N)":dbl}, "Result Out"=w3878:bool, "file error"=w3881:errorcluster)  [unwired: 10 in]
                    n2294 = local write "TEMP RISE LAB01-1"(w3876) -> ()
                    n2295 = local write "FAIL LAB01-1"(w3879) -> ()
                    n2296 = local write "DISP LAB01-1"(w3875) -> ()
                    n2297 = local write "RESULT LAB01-1"(w3878) -> ()
                    n2298 = local write "data file error"(w3881) -> ()
                  }
                }
              }
              frame #1 {
                # "LAB01-2"
                n2299 = case shown="True" w3891 {
                  tunnel: w3893 -> [_ w3906]
                  tunnel: w3890 -> [_ w3903]
                  tunnel: w3892 -> [_ w3902]
                  frame False {
                  }
                  frame True {
                    n2300 = local read "TEMP START LAB01-2"() -> (w3908:cluster{"TL":dbl, "TN":dbl})
                    n2301 = local read "FAIL LAB01-2"() -> (w3899:cluster{"LO":dbl, "HI":dbl})
                    n2302 = local read "TDMS LAB01-2"() -> (w3907:refnum<k34>)
                    n2303 = local read "SET LAB01-2"() -> (w3904:T5)
                    n2304 = local read "DISP LAB01-2"() -> (w3905:T4)
                    n2305 = local read "RESULT LAB01-2"() -> (w3896:bool)
                    n2306 = local read "SIG LAB01-2"() -> (w3909:T2)
                    n2307 = Bundle("FAIL LAB01-2"=w3899, "SIG LAB01-2"=w3909, "TEMP START LAB01-2"=w3908, "DISP LAB01-2"=w3905, "SET LAB01-2"=w3904, "TDMS LAB01-2"=w3907) -> (w3894:T29)  [unwired: 1 in]
                    n2308 = call "sub vi - cycle&temp fail v6.vi"("Amps Lo?"=w3906, "Input Cluster"=w3894, "SELECT"=w3903, "Amps Hi?"=w3902, "Result In"=w3896) -> ("(FAIL) out"=w3898:cluster{"FAIL LO":dbl, "FAIL HI":dbl}, "(DISP) out"=w3901:T4, "T-RISE"=w3895:cluster{"T-RISE (L)":dbl, "T-RISE (N)":dbl}, "Result Out"=w3897:bool, "file error"=w3900:errorcluster)  [unwired: 10 in]
                    n2309 = local write "TEMP RISE LAB01-2"(w3895) -> ()
                    n2310 = local write "FAIL LAB01-2"(w3898) -> ()
                    n2311 = local write "DISP LAB01-2"(w3901) -> ()
                    n2312 = local write "RESULT LAB01-2"(w3897) -> ()
                    n2313 = local write "data file error"(w3900) -> ()
                  }
                }
              }
              frame #2 {
                # "LAB02-1"
                n2314 = case shown="True" w3911 {
                  tunnel: w3913 -> [_ w3926]
                  tunnel: w3910 -> [_ w3923]
                  tunnel: w3912 -> [_ w3922]
                  frame False {
                  }
                  frame True {
                    n2315 = local read "TEMP START LAB02-1"() -> (w3928:cluster{"TL":dbl, "TN":dbl})
                    n2316 = local read "FAIL LAB02-1"() -> (w3919:cluster{"LO":dbl, "HI":dbl})
                    n2317 = local read "TDMS LAB02-1"() -> (w3927:refnum<k34>)
                    n2318 = local read "SET LAB02-1"() -> (w3924:T5)
                    n2319 = local read "DISP LAB02-1"() -> (w3925:T4)
                    n2320 = local read "SIG LAB02-1"() -> (w3929:T2)
                    n2321 = local read "RESULT LAB02-1"() -> (w3916:bool)
                    n2322 = Bundle("FAIL LAB02-1"=w3919, "SIG LAB02-1"=w3929, "TEMP START LAB02-1"=w3928, "DISP LAB02-1"=w3925, "SET LAB02-1"=w3924, "TDMS LAB02-1"=w3927) -> (w3914:T30)  [unwired: 1 in]
                    n2323 = call "sub vi - cycle&temp fail v6.vi"("Amps Lo?"=w3926, "Input Cluster"=w3914, "SELECT"=w3923, "Amps Hi?"=w3922, "Result In"=w3916) -> ("(FAIL) out"=w3918:cluster{"FAIL LO":dbl, "FAIL HI":dbl}, "(DISP) out"=w3921:T4, "T-RISE"=w3915:cluster{"T-RISE (L)":dbl, "T-RISE (N)":dbl}, "Result Out"=w3917:bool, "file error"=w3920:errorcluster)  [unwired: 10 in]
                    n2324 = local write "TEMP RISE LAB02-1"(w3915) -> ()
                    n2325 = local write "FAIL LAB02-1"(w3918) -> ()
                    n2326 = local write "DISP LAB02-1"(w3921) -> ()
                    n2327 = local write "RESULT LAB02-1"(w3917) -> ()
                    n2328 = local write "data file error"(w3920) -> ()
                  }
                }
              }
              frame #3 {
                # "LAB02-2"
                n2329 = case shown="True" w3931 {
                  tunnel: w3933 -> [_ w3946]
                  tunnel: w3930 -> [_ w3943]
                  tunnel: w3932 -> [_ w3942]
                  frame False {
                  }
                  frame True {
                    n2330 = local read "TEMP START LAB02-2"() -> (w3948:cluster{"TL":dbl, "TN":dbl})
                    n2331 = local read "FAIL LAB02-2"() -> (w3939:cluster{"LO":dbl, "HI":dbl})
                    n2332 = local read "TDMS LAB02-2"() -> (w3947:refnum<k34>)
                    n2333 = local read "SET LAB02-2"() -> (w3944:T5)
                    n2334 = local read "DISP LAB02-2"() -> (w3945:T4)
                    n2335 = local read "SIG LAB02-2"() -> (w3949:T2)
                    n2336 = local read "RESULT LAB02-2"() -> (w3936:bool)
